vi "Open 2601B.vi"(8 "错误输入（无错误）":errorcluster, 11 "数据保存":refnum<queue>) -> (0 "错误输出":errorcluster)   [LabVIEW 2021]
uses:
  VISA 2601B.vi
  LabView Lib/QueueLib/QueueLib.lvlib
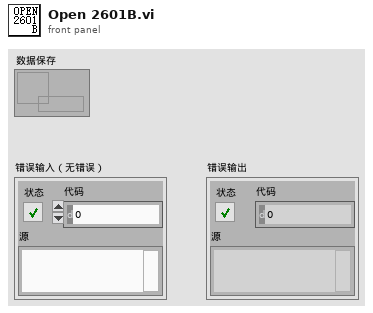
[diagram p1: front panel]
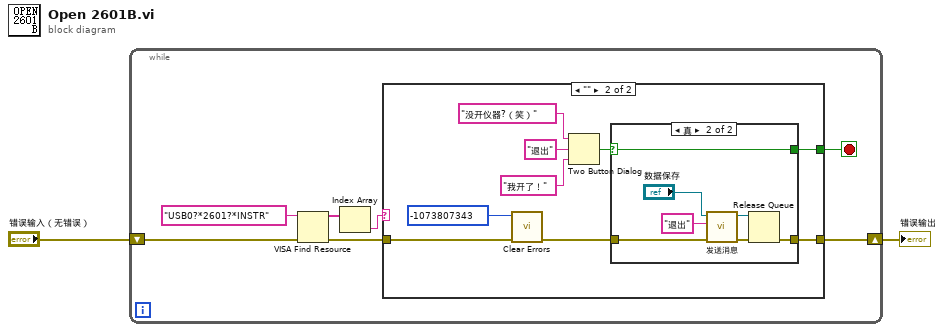
[diagram p0: block diagram]
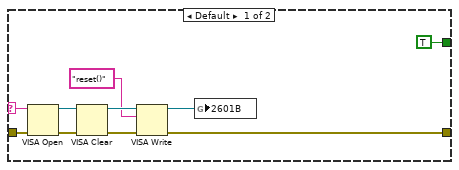
[diagram p2: hidden frame]
diagram:
  n1 = while {
    shift-right: [w9] -> w1
    shift-left: "错误输入（无错误）" -> [w8]
    stop <- w7 stop-if-true
    n2 = VISA Find Resource(8:w8, 11:"USB0?*2601?*INSTR" ("表达式(\"?*\")")) -> (0:w6:errorcluster, 3:w4:string[])  [unwired: 1 in, 1 out]
    n3 = Index Array(array=w4) -> (element=w3:string)  [unwired: 1 in]
    n4 = case shown="\"\"" w3 {
      selector: w3 -> [w11 _]
      tunnel: [w13 w24] -> w9
      tunnel: w6 -> [w14 w27]
      tunnel: [TRUE w22] -> w7
      frame Default {
        n5 = VISA Open(error in (no error)=w14, VISA resource name=w11) -> (VISA resource name=w19:refnum<visa-resource-name>, error out=w18:errorcluster)  [unwired: 3 in]
        n6 = VISA Clear(VISA resource name=w19, error in (no error)=w18) -> (VISA resource name out=w17:refnum<visa-resource-name>, error out=w16:errorcluster)
        n7 = VISA Write(VISA resource name=w17, write buffer="reset()" ("写入缓冲区"), error in (no error)=w16) -> (VISA resource name out=w10:refnum<visa-resource-name>, error out=w13:errorcluster)  [unwired: 1 out]
        n8 = global write "VISA 2601B.vi" "2601B"(w10) -> ()
      }
      frame "" {
        n9 = call <vilib>:"Clear Errors.vi"("error in (no error)"=w27, "specific error code to clear (0: all)"=-1073807343) -> ("error out"=w25:errorcluster)  [unwired: 4 in, 1 out]
        n10 = Two Button Dialog(message="没开仪器?（笑）" ("消息"), 1:"我开了！" ("T按钮名称（“确定”）"), 2:"退出" ("F按钮名称（“取消”）")) -> (T button?=w23:bool)
        n11 = case shown="真" w23 {
          selector: w23 -> [_ w34]
          tunnel: w25 -> [w29 w36]
          tunnel: [w29 w35] -> w24
          tunnel: [_ w34] -> w22
          frame False {
          }
          frame True {
            n12 = call-poly "发送消息.vi"("错误输入（无错误）"=w36, "消息"="退出", "输入队列"="数据保存") -> ("错误输出"=w32:errorcluster, "输出队列"=w31:refnum<queue>)  [unwired: 7 in]
            n13 = Release Queue(queue=w31, error in (no error)=w32) -> (error out=w35:errorcluster)  [unwired: 1 in, 2 out]
          }
        }
      }
    }
  }
  "错误输出" <- w1
